vi "Rabi Pulse Sequence Generator.vi"(5 "Optical Pulse":T1(array[cluster]), 7 "No. Instructions":i32, 8 "MW Delay":dbl, 9 "MW width step size":dbl=2e-09, 10 "MW width Max":dbl=5e-07, 11 "MW width Min":dbl=5e-08) -> (2 "Pulse Width":dbl[](array[numeric]), 3 "Pulse Sequence Out":T1(array[cluster]))   [LabVIEW 2012]
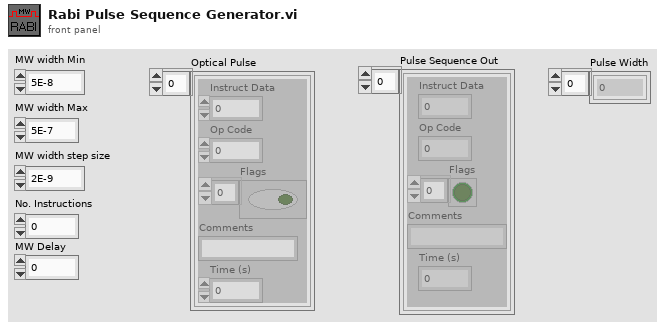
[diagram p1: front panel]
types:
  T1 = cluster{"Instruct Data":i32, "Op Code":i32, "Flags":bool[], "Comments":string, "Time (s)":dbl}[]
  T2 = cluster{"Instruct Data":i32, "Op Code":i32, "Flags":bool[], "Comments":string, "Time (s)":dbl}
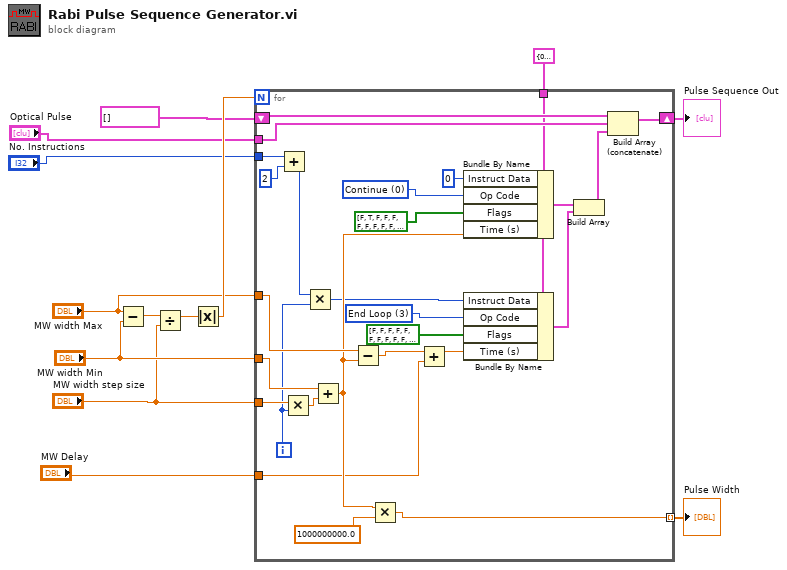
[diagram p0: block diagram]
diagram:
  n1 = Subtract(x="MW width Max", y="MW width Min") -> (x-y=w13:dbl)
  n2 = Divide(x=w13, y="MW width step size") -> (x/y=w12:dbl)
  n3 = Absolute Value(x=w12) -> (abs(x)=w11:dbl)
  n4 = for {
    N: w11 -> [_]
    shift-right: [w39] -> w2
    shift-left: T1 [] -> [w40]
    tunnel: "Optical Pulse" -> [w37]
    tunnel: T2 {"Instruct Data"=0, "Op Code"=0, "Flags"=[FALSE, FALSE, FALSE, FALSE, FALSE, FALSE, FALSE, FALSE, FALSE, FALSE, FALSE, FALSE, FALSE, FALSE, FALSE, FALSE, FALSE, FALSE, FALSE, FALSE, FALSE, TRUE, TRUE, TRUE], "Comments"="", "Time (s)"=0.01} ("PB Inst 2") -> [w29]
    tunnel: "MW width Min" -> [w28]
    tunnel: "MW width step size" -> [w33]
    tunnel: "MW width Max" -> [w26]
    tunnel: "MW Delay" -> [w16]
    tunnel: [w15] -> w3 mode=indexing
    tunnel: "No. Instructions" -> [w14]
    i -> [w22]
    w30 = 3 items=["Continue", "Stop", "Loop", "End Loop", "JSR", "RTS", "Branch", "Long Delay", "Wait"] ("Op Code")
    w35 = 0 items=["Continue", "Stop", "Loop", "End Loop", "JSR", "RTS", "Branch", "Long Delay", "Wait"] ("Op Code")
    n5 = Add(x=w14, y=2) -> (x+y=w23:i32)
    n6 = Multiply(x=w33, y=w22) -> (x*y=w32:dbl)
    n7 = Multiply(x=w23, y=w22) -> (x*y=w21:i32)
    n8 = Add(x=w28, y=w32) -> (x+y=w25:dbl)
    n9 = Subtract(x=w26, y=w25) -> (x-y=w27:dbl)
    n10 = Multiply(x=w25, y=1000000000.0) -> (x*y=w15:dbl)
    n11 = Add(x=w27, y=w16) -> (x+y=w17:dbl)
    n12 = Bundle By Name(cluster=w29, "Instruct Data"=0, "Op Code"=w35, "Flags"=bool[] [FALSE, TRUE, FALSE, FALSE, FALSE, FALSE, FALSE, FALSE, FALSE, FALSE, FALSE, FALSE, FALSE, FALSE, FALSE, FALSE, FALSE, FALSE, FALSE, FALSE, FALSE, TRUE, TRUE, TRUE], "Time (s)"=w25) -> (w20:T2)
    n13 = Bundle By Name(cluster=w29, "Instruct Data"=w21, "Op Code"=w30, "Flags"=bool[] [FALSE, FALSE, FALSE, FALSE, FALSE, FALSE, FALSE, FALSE, FALSE, FALSE, FALSE, FALSE, FALSE, FALSE, FALSE, FALSE, FALSE, FALSE, FALSE, FALSE, FALSE, TRUE, TRUE, TRUE], "Time (s)"=w17) -> (w19:T2)
    n14 = Build Array(w20, w19) -> (w18:T1)
    n15 = Build Array (concatenate)(w40, w37, w18) -> (w39:T1)
  }
  "Pulse Width" <- w3
  "Pulse Sequence Out" <- w2
